vi "Read RequirementsMap.vi"(11 "TraceabilityMatrix in":refnum<class "TraceabilityMatrix.lvclass">) -> (2 "RequirementMap":map{string, set{string}}(c390), 3 "TraceabilityMatrix out":refnum<class "TraceabilityMatrix.lvclass">)   [LabVIEW 2021, in "Bananas.lvlib" / "TraceabilityMatrix.lvclass"]
uses:
  TraceabilityMatrix.lvclass
  TraceabilityMatrix.lvclass/TraceabilityMatrix.ctl
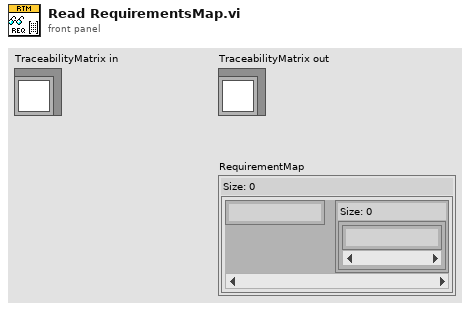
[diagram p1: front panel]
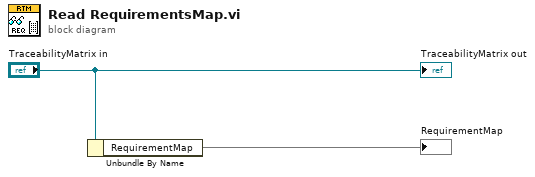
[diagram p0: block diagram]
diagram:
  n1 = Unbundle By Name("TraceabilityMatrix in") -> ("RequirementMap"=→"RequirementMap":map{string, set{string}})
  "TraceabilityMatrix out" <- "TraceabilityMatrix in"
